vi "Get Channel Names and Default Values.vi"(8 "error in":errorcluster, 10 "channels":refnum<class "Channel.lvclass">[](array[class]), 11 "digital output mode in":refnum<class "Digital Output Mode.lvclass">) -> (0 "error out":errorcluster, 1 "default values":dbl[](array[numeric]), 2 "names":string[](array[string]), 3 "digital output mode out":refnum<class "Digital Output Mode.lvclass">)   [LabVIEW 2017, in "Scan Engine Scripting.lvlib" / "Digital Output Mode.lvclass"]
uses:
  Digital Output Mode.lvclass
  Channel Classes/Channel/Channel.lvclass
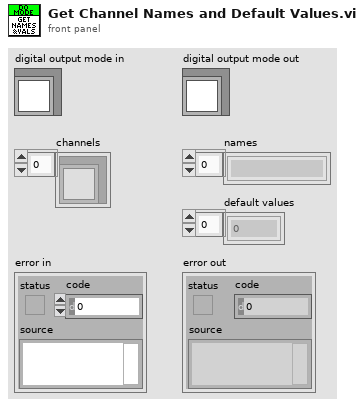
[diagram p1: front panel]
types:
  T1 = typedef "Scan Engine Scripting.lvlib/digital channel settings.ctl" = cluster{"name":string, "default value":bool}
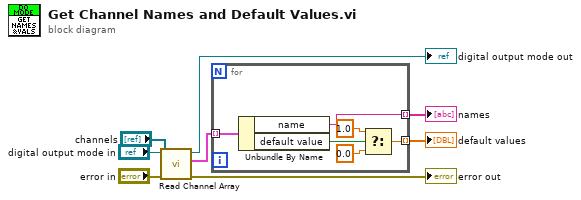
[diagram p0: block diagram]
diagram:
  n1 = call "Read Channel Array.vi"("error in"="error in", "channels"="channels", "digital output mode in"="digital output mode in") -> ("error out"=→"error out":errorcluster, "channel settings"=w7:T1[], "digital output mode out"=→"digital output mode out":refnum<class "Digital Output Mode.lvclass">)  [unwired: 6 in]
  n2 = for {
    tunnel: w7 -> [w14] mode=indexing
    tunnel: [w13] -> w3 mode=indexing
    tunnel: [w9] -> w2 mode=indexing
    n3 = Unbundle By Name(w14) -> ("name"=w13:string, "default value"=w12:bool)
    n4 = Select(t=1.0, s=w12, f=0.0) -> (s? t:f=w9:dbl)
  }
  "names" <- w3
  "default values" <- w2
